vi "Build Synchronous Message with Arguments.vi"(5 "State with Arguments":string, 7 "Arguments (\"\")":string, 9 "Target Module (\"\")":string) -> (6 "State with Arguments out":string)   [LabVIEW 2020, in "Communicable State Machine.lvlib"]
doc: "Builds a message that contains arguments for CSM. This VI will parse \"State with Arguments\" for message string, arguments and target module from input <b>State with Arguments</b> and replace corresponding parts in the message with input values with sync-message symobol \"-@\" if <b>Target Module (\"\")</b> is specified.\n\n<B>For Example:</B>\n\nIf <b>State with Arguments</b> input is \"API: DoSth\"\n<b>Arguments (\"\")</b> input is \"Arguments\"\n<b>Target Module (\"\")</b> input is \"Callee\"\nThen result string is \"API: DoSth >> Arguments ->| Callee\". It's different with Build Message with Arguments(Auto Check).vi. Message Type Symbol is replaced with \"-@\".\n\nIf <b>State with Arguments</b> input is \"API: DoSth >> Arguments -> Callee\"\n<b>Arguments (\"\")</b> input is \"NewArguments\"\n<b>Target Module (\"\")</b> input is \"\"\nThen result string is \"API: DoSth >> NewArguments ->| Callee\". Message Type Symbol is replaced with \"-@\".\n\nIf <b>State with Arguments</b> input is \"API: DoSth >> Arguments -> Callee\"\n<b>Arguments (\"\")</b> input is \"NewArguments\"\n<b>Target Module (\"\")</b> input is \"NewCallee\"\nThen result string is \"API: DoSth >> NewArguments -@ NewCallee\". Message Type Symbol is replaced with \"-@\".\n\nIf <b>State with Arguments</b> input is \"API: DoSth >> Arguments -> Callee\"\n<b>Arguments (\"\")</b> input is \"\"\n<b>Target Module (\"\")</b> input is \"NewCallee\"\nThen result string is \"API: DoSth -@ NewCallee\". Message Type Symbol is replaced with \"-@\".\n\nIf <b>State with Arguments</b> input is \"API: DoSth >> Arguments -@ Callee\"\n<b>Arguments (\"\")</b> input is \"NewArguments\"\n<b>Target Module (\"\")</b> input is \"\"\nThen result string is \"API: DoSth >> NewArguments -@ Callee\".\n\n<b>Inputs:</b>\n - <b>State with Arguments</b>: Input Message which might contain Arguments or target Module\n - <b>Arguments (\"\")</b>: The arguments which will be used to replace arguments in <b>State with Arguments</b>. if empty, no arguments will be included in output strings.\n - <b>Target Module (\"\")</b>: The target which will be used to replace target in <b>State with Arguments</b>. if empty, target in <b>State with Arguments</b> will be used.\n\n<b>Outputs:</b>\n - <b>State with Arguments</b>: String stands for state with arguments"
uses:
  Communicable State Machine.lvlib
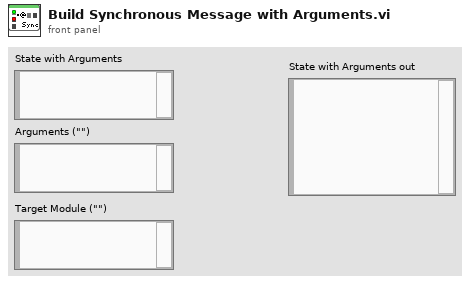
[diagram p1: front panel]
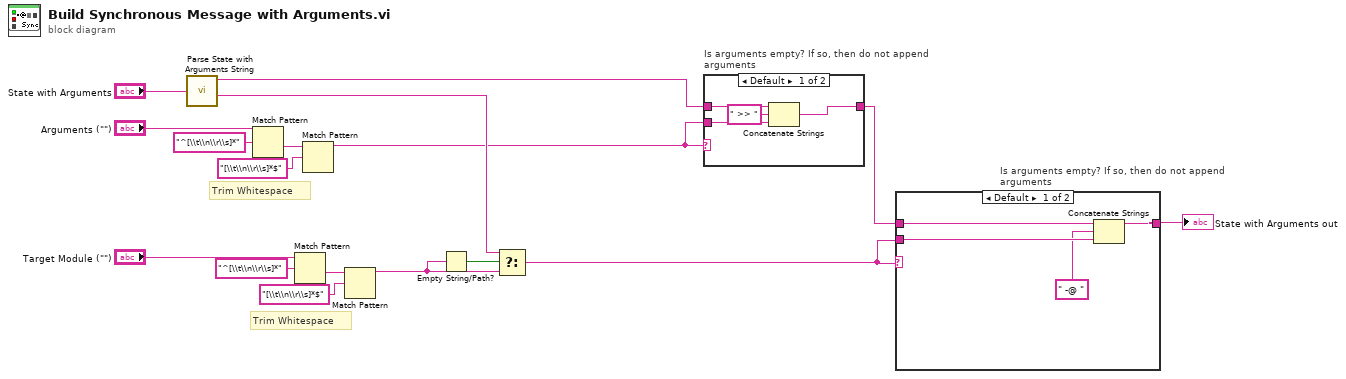
[diagram p0: block diagram]
diagram:
  # "Trim Whitespace"
  # "Trim Whitespace"
  n1 = call "Parse State with Arguments String.vi"("State with Arguments"="State with Arguments") -> ("State"=w5:string, "Target Module"=w8:string)  [unwired: 6 in, 2 out]
  n2 = Match Pattern(string="Arguments (\"\")", regular expression="^[\\t\\n\\r\\s]*") -> (after substring=w14:string)  [unwired: 1 in, 3 out]
  n3 = Match Pattern(string="Target Module (\"\")", regular expression="^[\\t\\n\\r\\s]*") -> (after substring=w11:string)  [unwired: 1 in, 3 out]
  n4 = Match Pattern(string=w14, regular expression="[\\t\\n\\r\\s]*$") -> (before substring=w1:string)  [unwired: 1 in, 3 out]
  n5 = Match Pattern(string=w11, regular expression="[\\t\\n\\r\\s]*$") -> (before substring=w7:string)  [unwired: 1 in, 3 out]
  n6 = Empty String/Path?(string/path=w7) -> (empty?=w9:bool)
  n7 = Select(t=w8, s=w9, f=w7) -> (s? t:f=w2:string)
  n8 = case "Is arguments empty? If so, then do not append arguments" shown="Default" w1 {
    tunnel: [w18 w22] -> w16
    tunnel: w5 -> [w21 w22]
    tunnel: w1 -> [w19 _]
    frame Default {
      n9 = Concatenate Strings(w21, " >> " ("string"), w19) -> (w18:string)
    }
    frame "" {
    }
  }
  n10 = case "Is arguments empty? If so, then do not append arguments" shown="Default" w2 {
    tunnel: [w24 w27] -> w17
    tunnel: w16 -> [w26 w27]
    tunnel: w2 -> [w25 _]
    frame Default {
      n11 = Concatenate Strings(w26, " -@ " ("string"), w25) -> (w24:string)
    }
    frame "" {
    }
  }
  "State with Arguments out" <- w17
